vi "load_class.vi"(7 "config in":T1, 8 "error in (no error)":errorcluster, 10 "commit_hash":string, 11 "lvclass_path":path) -> (0 "error out":errorcluster, 2 "config out":T1, 3 "lv-builder":refnum<class "lv-builder.lvclass">)   [LabVIEW 2015, in "lv-build-interface.lvlib"]
uses:
  lv-build-interface.lvlib
  lv-build/public/_controls/configuration.ctl
  lv-builder/class/lv-builder.lvclass
  lv-builder/lv-builder.lvlib
  lv-build/lv-build.lvlib
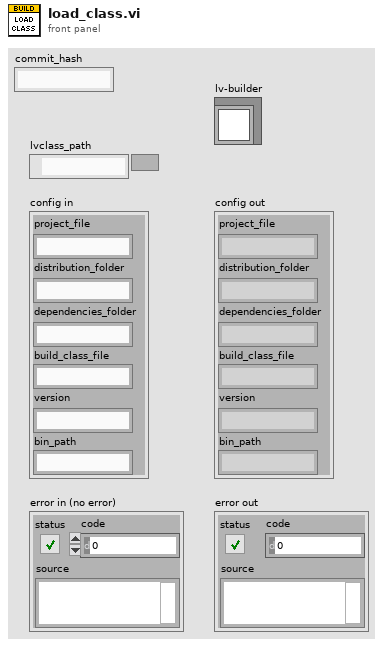
[diagram p1: front panel]
types:
  T1 = typedef "lv-build.lvlib/configuration.ctl" = cluster{"project_file":string, "distribution_folder":string, "dependencies_folder":string, "build_class_file":string, "version":string, "bin_path":string}
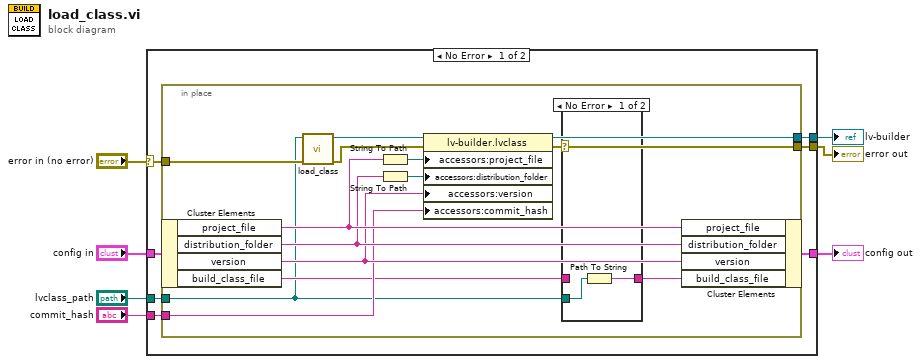
[diagram p0: block diagram]
diagram:
  n1 = case shown="No Error" "error in (no error)" {
    selector: "error in (no error)" -> [w14 w33]
    tunnel: "config in" -> [w9 w32]
    tunnel: [w13 _] -> w5
    tunnel: [w10 w32] -> w4
    tunnel: "lvclass_path" -> [w12 _]
    tunnel: [w11 w33] -> w2
    tunnel: "commit_hash" -> [w8 _]
    frame No Error {
      n2 = in-place {
        in-place-border: w14 -> [w28]
        in-place-border: [w26] -> w13
        in-place-border: w12 -> [w15]
        in-place-border: [w18] -> w11
        in-place-border: w8 -> [w19]
        n3 = in-place-cluster #1(w9) -> ("project_file"=w22:string, "distribution_folder"=w21:string, "version"=w20:string, "build_class_file"=w17:string)
        n4 = call "load_class.vi"("error in (no error)"=w28, "class"=w15) -> ("error out"=w25:errorcluster, "lv_build_plugin"=w27:refnum<class "lv-builder.lvclass">)  [unwired: 8 in]
        n5 = String To Path(string=w22) -> (path=w23:path)
        n6 = String To Path(string=w21) -> (path=w24:path)
        n7 = property class="lv-builder.lvclass"(reference=w27, error in=w25, "accessors:project_file"=w23, "accessors:distribution_folder"=w24, "accessors:version"=w20, "accessors:commit_hash"=w19) -> (reference out=w26:refnum<class "lv-builder.lvclass">, error out=w18:errorcluster)
        n8 = case shown="No Error" w18 {
          tunnel: w15 -> [w29 _]
          tunnel: w17 -> [_ w31]
          tunnel: [w30 w31] -> w16
          frame No Error {
            n9 = Path To String(path=w29) -> (string=w30:string)
          }
          frame Error {
          }
        }
        n10 = in-place-cluster #1("project_file"=w22, "distribution_folder"=w21, "version"=w20, "build_class_file"=w16) -> (w10:T1)
      }
    }
    frame Error {
    }
  }
  "lv-builder" <- w5
  "config out" <- w4
  "error out" <- w2
